vi "DCR3 Lamp.vi"() -> ()   [LabVIEW 2012]
uses:
  <vilib>/Instr/_visa.llb/VISA Configure Serial Port (Instr).vi
panel:
  in  "Case Constant\n(See Context Help)":bool=TRUE
  out "Firmware Version":string
  in  "delay before read (ms)":u32=500
  in  "read":bool=TRUE
  in  "string to write":string="*IDN?\r\n"
  in  "write":bool=TRUE
  out "bytes read":u32
  out "read string":string
  in  "VISA resource name":refnum<visa-resource-name>="COM1"
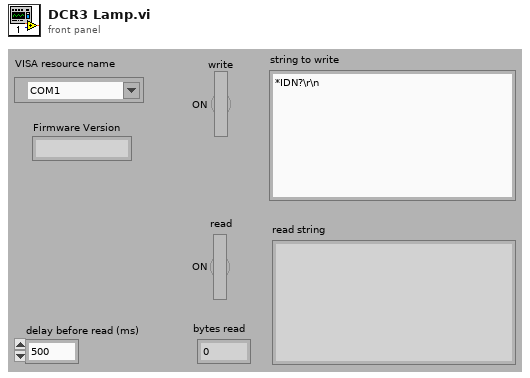
[diagram p1: front panel]
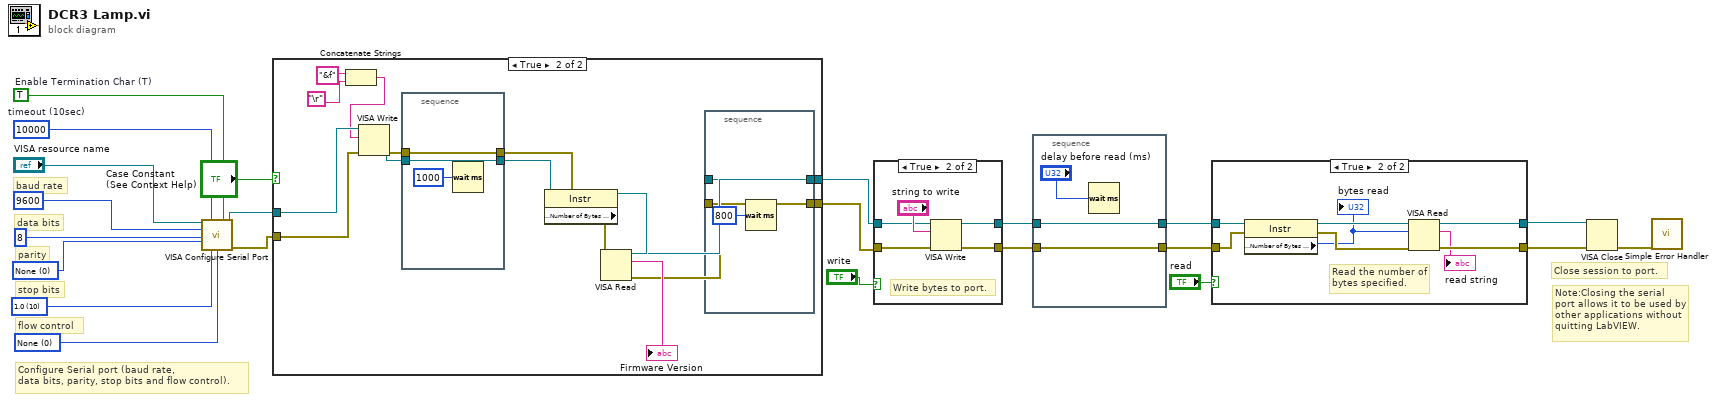
[diagram p0: block diagram]
diagram:
  w6 = u16 0 items=["None"=0, "XON/XOFF"=1, "RTS/CTS"=2, "DTR/DSR"=4] ("flow control")
  w7 = u16 10 items=["1.0"=10, "1.5"=15, "2.0"=20] ("stop bits")
  w8 = u16 0 items=["None", "Odd", "Even", "Mark", "Space"] ("parity")
  w16 = TRUE  # Enable Termination Char (T)
  w17 = u32 10000  # timeout (10sec)
  # "flow control"
  # "stop bits"
  # "parity"
  # "data bits"
  # "baud rate"
  # "Note:Closing the serial port allows it to be used by other applications without\nquitting LabVIEW."
  # "Configure Serial port (baud rate,\ndata bits, parity, stop bits and flow control)."
  # "Close session to port."
  n1 = call-poly "VISA Configure Serial Port"("VISA resource name"="VISA resource name", "timeout (10sec)"=w17, "Enable Termination\nChar (T)"=w16, "baud rate (9600)"=u32 9600 ("baud rate"), "data bits (8)"=u16 8 ("data bits"), "parity (0:none)"=w8, "stop bits (10: 1 bit)"=w7, "flow control (0:none)"=w6) -> ("VISA resource name out"=w5:refnum<visa-resource-name>, "error out"=w4:errorcluster)  [unwired: 6 in]
  n2 = case shown="True" "Case Constant\n(See Context Help)" {
    tunnel: w5 -> [w24 w37]
    tunnel: w4 -> [w23 w36]
    tunnel: [w24 w31] -> w3
    tunnel: [w23 w30] -> w2
    frame False {
    }
    frame True {
      n3 = Concatenate Strings("&f" ("write buffer"), "\r") -> (w25:string)
      n4 = VISA Write(VISA resource name=w37, write buffer=w25, error in (no error)=w36) -> (VISA resource name out=w28:refnum<visa-resource-name>, error out=w29:errorcluster)  [unwired: 1 out]
      n5 = stacked-sequence {
        tunnel: [w40] -> _
        tunnel: w29 -> [w40]
        tunnel: [w39] -> _
        tunnel: w28 -> [w39]
        frame #0 {
          n6 = Wait (ms)(milliseconds to wait=u32 1000) -> ()  [unwired: 1 out]
        }
      }
      n7 = property class="Instr"(reference=w28, error in=w29) -> (reference out=w35:refnum<visa-resource-name>, error out=w34:errorcluster, "Serial Settings:Number of Bytes at Serial Port"=w33:u32)
      n8 = VISA Read(VISA resource name=w35, byte count=w33, error in (no error)=w34) -> (VISA resource name out=w31:refnum<visa-resource-name>, read buffer=→"Firmware Version":string, error out=w30:errorcluster)  [unwired: 1 out]
      n9 = stacked-sequence {
        tunnel: [w42] -> _
        tunnel: w31 -> [w42]
        tunnel: [w41] -> _
        tunnel: w30 -> [w41]
        frame #0 {
          n10 = Wait (ms)(milliseconds to wait=u32 800) -> ()  [unwired: 1 out]
        }
      }
    }
  }
  n11 = case shown="True" "write" {
    tunnel: [w45 w50] -> w14
    tunnel: w3 -> [w44 w48]
    tunnel: w2 -> [w45 w47]
    tunnel: [w44 w46] -> w12
    frame False {
    }
    frame True {
      # "Write bytes to port."
      n12 = VISA Write(VISA resource name=w48, write buffer="string to write", error in (no error)=w47) -> (VISA resource name out=w46:refnum<visa-resource-name>, error out=w50:errorcluster)  [unwired: 1 out]
    }
  }
  n13 = stacked-sequence {
    tunnel: w14 -> [w53]
    tunnel: [w53] -> w13
    tunnel: w12 -> [w52]
    tunnel: [w52] -> w11
    frame #0 {
      n14 = Wait (ms)(milliseconds to wait="delay before read (ms)") -> ()  [unwired: 1 out]
    }
  }
  n15 = case shown="True" "read" {
    tunnel: w13 -> [w55 w59]
    tunnel: [w55 w63] -> w20
    tunnel: [w54 w62] -> w19
    tunnel: w11 -> [w54 w61]
    frame False {
    }
    frame True {
      # "Read the number of bytes specified."
      n16 = property class="Instr"(reference=w61, error in=w59) -> (reference out=w60:refnum<visa-resource-name>, error out=w58:errorcluster, "Serial Settings:Number of Bytes at Serial Port"=w56:u32)
      "bytes read" <- w56
      n17 = VISA Read(VISA resource name=w60, byte count=w56, error in (no error)=w58) -> (VISA resource name out=w62:refnum<visa-resource-name>, read buffer=→"read string":string, error out=w63:errorcluster)  [unwired: 1 out]
    }
  }
  n18 = VISA Close(VISA resource name=w19, error in (no error)=w20) -> (error out=w18:errorcluster)
  n19 = call <vilib>:"Simple Error Handler.vi"("error in (no error)"=w18) -> ()  [unwired: 4 in, 5 out]
